vi "lockin time constant.vi"() -> (0 "appended array":string[][](array[string]))   [LabVIEW 2010]
panel:
  out "Response":string
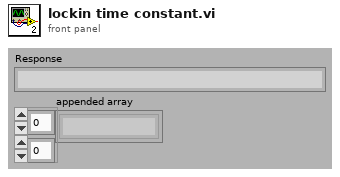
[diagram p1: front panel]
types:
  T1 = enum16{"Set Amplitude", "Get Amplitude", "Set Frequency", "Get Frequency", "Set Harmonic", "Get Harmonic", "Set Phase", "Get Phase", "Auto Phase", "Add to Phase", "Autogain", "Set Time Constant", "Get Time Constant", "Set Sensitivity", "Get Sensitivity", "Set Input A", "Set Input A-B", "Get Input Setting", "Set Offset", "Get Offset"}
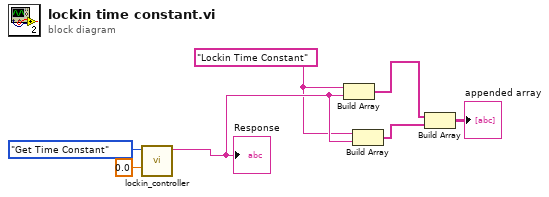
[diagram p0: block diagram]
diagram:
  w4 = "Lockin Time Constant" ("element")
  n1 = call "lockin_controller.vi"("Numerical Argument"=0.0, "Command"=T1."Get Time Constant") -> ("Response"=w5:string)  [unwired: 9 in]
  "Response" <- w5
  n2 = Build Array(w4, w5) -> (w2:string[])
  n3 = Build Array(w4, w5) -> (w3:string[])
  n4 = Build Array(w2, w3) -> (→"appended array":string[][])
